vi "AddHiddenDevice.vi"(2 "error in (no error)":errorcluster, 3 "DeviceToHide":string, 4 "SetListPrefs in":refnum<class "SetListPrefs.lvclass">) -> (0 "error out":errorcluster, 1 "SetListPrefs out":refnum<class "SetListPrefs.lvclass">)   [LabVIEW 2013, in "SetListPrefs.lvclass"]
uses:
  SetListPrefs.lvclass
  SetListPrefs.lvclass/SetListPrefs.ctl
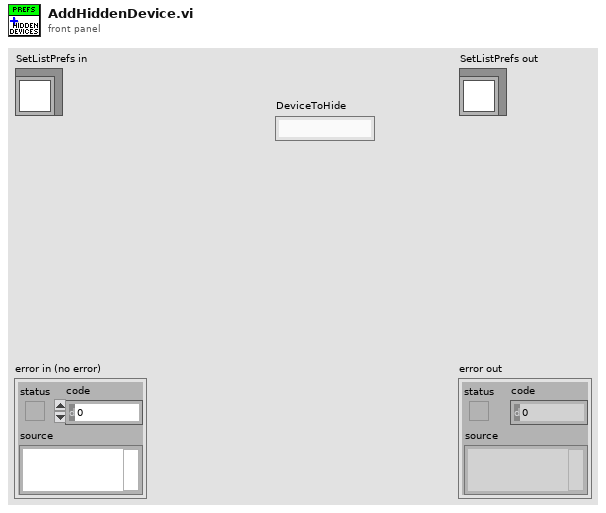
[diagram p1: front panel]
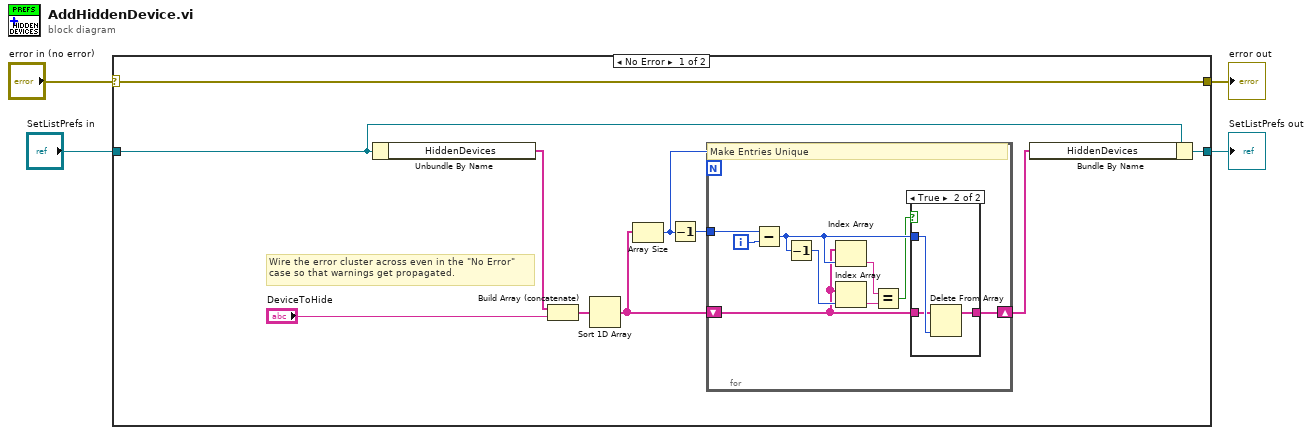
[diagram p0: block diagram]
diagram:
  n1 = case shown="No Error" "error in (no error)" {
    selector: "error in (no error)" -> [w14 w29]
    tunnel: [w14 w29] -> w3
    tunnel: [w5 w28] -> w1
    tunnel: "SetListPrefs in" -> [w6 w28]
    frame No Error {
      # "Wire the error cluster across even in the \"No Error\"\ncase so that warnings get propagated."
      n2 = Unbundle By Name(w6) -> ("HiddenDevices"=w7:string[])
      n3 = Build Array (concatenate)(w7, "DeviceToHide") -> (w9:string[])
      n4 = Sort 1D Array(array=w9) -> (sorted array=w11:string[])
      n5 = Array Size(array=w11) -> (size(s)=w10:i32)
      n6 = Decrement(x=w10) -> (x-1=w12:i32)
      n7 = for {
        N: w10 -> [_]
        shift-right: [w16] -> w13
        shift-left: w11 -> [w17]
        tunnel: w12 -> [w23]
        i -> [w22]
        # "Make Entries Unique"
        n8 = Subtract(x=w23, y=w22) -> (x-y=w18:i32)
        n9 = Decrement(x=w18) -> (x-1=w19:i32)
        n10 = Index Array(array=w17, index=w18) -> (element=w21:string)
        n11 = Index Array(array=w17, index=w19) -> (element=w20:string)
        n12 = Equal?(x=w21, y=w20) -> (x = y?=w15:bool)
        n13 = case shown="True" w15 {
          tunnel: w18 -> [_ w27]
          tunnel: w17 -> [w24 w26]
          tunnel: [w24 w25] -> w16
          frame False {
          }
          frame True {
            n14 = Delete From Array(array=w26, index=w27) -> (array with subset deleted=w25:string[])  [unwired: 1 in, 1 out]
          }
        }
      }
      n15 = Bundle By Name(cluster=w6, "HiddenDevices"=w13) -> (w5:refnum<class "SetListPrefs.lvclass">)
    }
    frame Error {
    }
  }
  "error out" <- w3
  "SetListPrefs out" <- w1
